vi "Count Result by Type.vi"(8 "error in (no error)":errorcluster, 10 "Result Type":T1, 11 "Mock Result Observer In":refnum<class "Mock Result Observer.lvclass">) -> (0 "error out":errorcluster, 2 "Numeric":i32, 3 "Mock Result Observer Out":refnum<class "Mock Result Observer.lvclass">)   [LabVIEW 2020, in "Mock Result Observer.lvclass"]
uses:
  Mock Result Observer.lvclass
  source/Core/Result/Type.ctl
  source/Core/Result/Result.lvlib
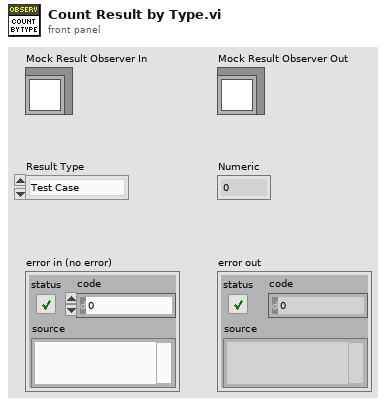
[diagram p1: front panel]
types:
  T1 = typedef "Result.lvlib/Type.ctl" = enum16{"Test Case", "Test Suite", "Test Run", "Pass", "Fail", "Skip", "Pass if", "Fail if", "Pass if Error", "Fail if Error", "Pass if Equal", "Fail if Equal"}
  T2 = typedef "Result.lvlib/Result.ctl" = cluster{"Name":string, "Description":string, "Status":T3, "Result Type":T1, "Execution Time":dbl, "Data":cluster{"Expected":variant, "Actual":variant, "Delta":variant}}
  T3 = typedef "Result.lvlib/Status.ctl" = enum16{"", "Passed", "Failed", "Error", "Skipped", "Setup Error", "Broken", "Teardown Error"}
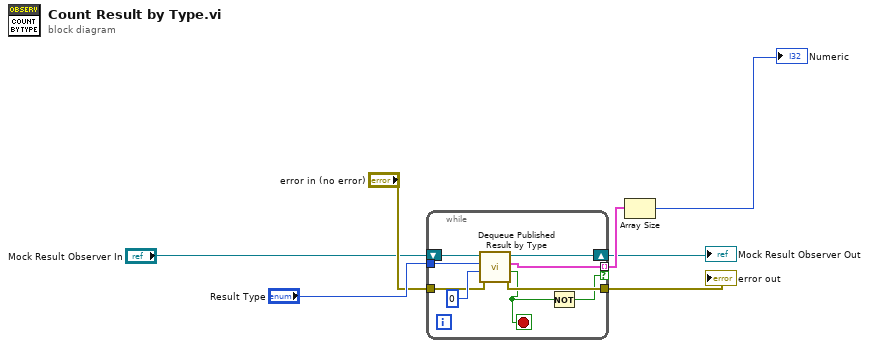
[diagram p0: block diagram]
diagram:
  n1 = while {
    tunnel: "error in (no error)" -> [w14]
    tunnel: "Result Type" -> [w12]
    shift-right: [w13] -> w3
    shift-left: "Mock Result Observer In" -> [w15]
    tunnel: [w11] -> w5
    tunnel: [w10] -> w6 mode=indexing if=w8
    stop <- w9 stop-if-true
    n2 = call "Dequeue Published Result by Type.vi"("error in (no error)"=w14, "timeout in ms"=0, "Result Type"=w12, "Mock Result Observer In"=w15) -> ("error out"=w11:errorcluster, "timed out?"=w9:bool, "Result"=w10:T2, "Mock Result Observer Out"=w13:refnum<class "Mock Result Observer.lvclass">)  [unwired: 4 in]
    n3 = Not(x=w9) -> (.not. x?=w8:bool)
  }
  "error out" <- w5
  "Mock Result Observer Out" <- w3
  n4 = Array Size(array=w6) -> (size(s)=→"Numeric":i32)
